vi "Format AI DAQ Configuration Log.vi"(8 "error in (no error)":errorcluster, 11 "Instrument.Lockin in":refnum<class "Instrument.Lockin.lvclass">) -> (0 "error out":errorcluster, 2 "Array":T1[](array[typedef]), 3 "Instrument.Lockin out":refnum<class "Instrument.Lockin.lvclass">)   [LabVIEW 2019, in "Instrument.Lockin.lvlib" / "Instrument.Lockin.lvclass"]
uses:
  Instrument.Lockin.lvclass
  Typedefs/Lockin.LogConfiguration.DAQ--Cluster.ctl
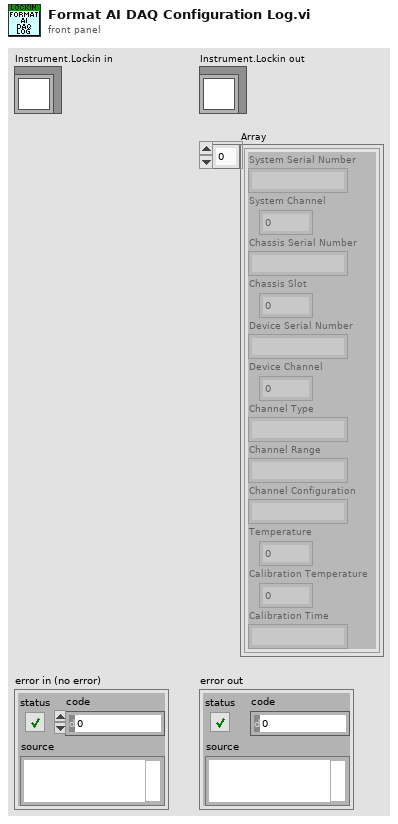
[diagram p1: front panel]
types:
  T1 = typedef "Instrument.Lockin.lvlib/Instrument.Lockin.lvclass/Lockin.LogConfiguration.DAQ--Cluster.ctl" = cluster{"System Serial Number":string, "System Channel":i32, "Chassis Serial Number":string, "Chassis Slot":i32, "Device Serial Number":string, "Device Channel":i32, "Channel Type":string, "Channel Range":string, "Channel Configuration":string, "Temperature":dbl, "Calibration Temperature":dbl, "Calibration Time":string}
  T2 = typedef "Instrument.Lockin.lvlib/Instrument.DAQ.lvclass/AI.Channel--Cluster--Array.ctl" = T3[]
  T3 = typedef "Instrument.Lockin.lvlib/Instrument.DAQ.lvclass/AI.Channel--Cluster.ctl" = cluster{"Enable?":bool, "Channel":i32, "References":u16[], "reference index":i32}
  T4 = typedef "Instrument.Lockin.lvlib/Instrument.DAQ.lvclass/DeviceInfo--Cluster.ctl" = cluster{"DeviceName":string, "DevIsSimulated":bool, "DeviceSerialNumber":string, "ProductType":string, "ProductCategory":i32, "ProductNumber":u32, "ChassisNumber":u32, "SlotNumber":u32, "ChassisName":string, "ChassisSerialNumber":string, "DevTemp":dbl, "SelfCal.LastDate/Time":string, "SelfCal.LastTemp":dbl, "calibration due?":bool}
  T5 = typedef "Instrument.Lockin.lvlib/Instrument.DAQ.lvclass/DAQ.Config.AI--Cluster--Array.ctl" = cluster{"Channels":tag, "Coupling":T6, "Range":T7, "terminal configuration":T8, "Type":T9}[]
  T6 = typedef "Instrument.Lockin.lvlib/Instrument.DAQ.lvclass/DAQ.Config.AI.Coupling--enum.ctl" = u16
  T7 = typedef "Instrument.Lockin.lvlib/Instrument.DAQ.lvclass/DAQ.Config.AI.Range--enum.ctl" = enum16{"±0.316", "±1.00", "±3.16", "±10.0", "±31.6", "±42.4", ""}
  T8 = typedef "Instrument.Lockin.lvlib/Instrument.DAQ.lvclass/DAQ.TerminalConfiguration--ring.ctl" = i32
  T9 = typedef "Instrument.Lockin.lvlib/Instrument.DAQ.lvclass/DAQ.Type--enum.ctl" = enum16{"None", "USB-4431", "PXI-446x"}
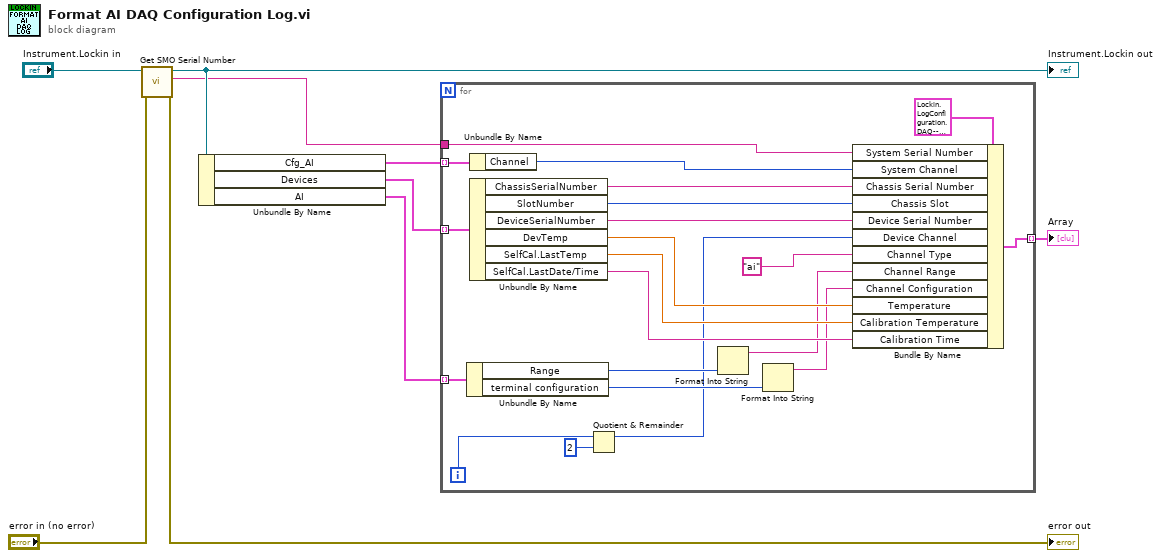
[diagram p0: block diagram]
diagram:
  n1 = call-dynamic "Get SMO Serial Number.vi"("error in (no error)"="error in (no error)", "Instrument.Lockin in"="Instrument.Lockin in") -> ("error out"=→"error out":errorcluster, "Serial Number"=w7:string, "Instrument.Lockin out"=w9:refnum<class "Instrument.Lockin.lvclass">)  [unwired: 7 in]
  "Instrument.Lockin out" <- w9
  n2 = Unbundle By Name(w9) -> ("Cfg_AI"=w4:T2, "Devices"=w5:T4[], "AI"=w6:T5)
  n3 = for {
    tunnel: [w30] -> w2 mode=indexing
    tunnel: w7 -> [w13]
    tunnel: w5 -> [w28] mode=indexing
    tunnel: w4 -> [w27] mode=indexing
    tunnel: w6 -> [w19] mode=indexing
    i -> [w12]
    n4 = Unbundle By Name(w19) -> ("Range"=w18:T7, "terminal configuration"=w15:T8)
    n5 = Unbundle By Name(w27) -> ("Channel"=w26:i32)
    n6 = Unbundle By Name(w28) -> ("ChassisSerialNumber"=w25:string, "SlotNumber"=w24:u32, "DeviceSerialNumber"=w23:string, "DevTemp"=w20:dbl, "SelfCal.LastTemp"=w21:dbl, "SelfCal.LastDate/Time"=w22:string)
    n7 = Quotient & Remainder(x=w12, y=2) -> (x-y*floor(x/y)=w10:i32)  [unwired: 1 out]
    n8 = Format Into String(w18) -> (resulting string=w17:string)  [unwired: 3 in, 1 out]
    n9 = Format Into String(w15) -> (resulting string=w16:string)  [unwired: 3 in, 1 out]
    n10 = Bundle By Name(cluster=T1 {"System Serial Number"="", "System Channel"=0, "Chassis Serial Number"="", "Chassis Slot"=0, "Device Serial Number"="", "Device Channel"=0, "Channel Type"="", "Channel Range"="", "Channel Configuration"="", "Temperature"=0.0, "Calibration Temperature"=0.0, "Calibration Time"=""} ("DAQ Configuration"), "System Serial Number"=w13, "System Channel"=w26, "Chassis Serial Number"=w25, "Chassis Slot"=w24, "Device Serial Number"=w23, "Device Channel"=w10, "Channel Type"="ai" ("format string"), "Channel Range"=w17, "Channel Configuration"=w16, "Temperature"=w20, "Calibration Temperature"=w21, "Calibration Time"=w22) -> (w30:T1)
  }
  "Array" <- w2
